vi "Open and close new editor.vi"(8 "error in (no error)":errorcluster) -> (0 "error out":errorcluster)   [LabVIEW 2013]
doc: "This vi is used to close 'Add device' editor and open 'Edit device' editor after adding device to database."
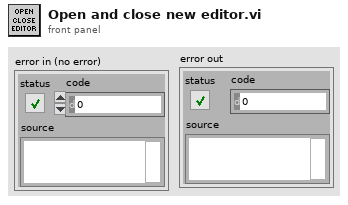
[diagram p1: front panel]
types:
  T1 = enum32{"invalid app kind", "Development System", "Run Time System", "Student Edition", "Embedded LabVIEW", "Evaluation", "Custom"}
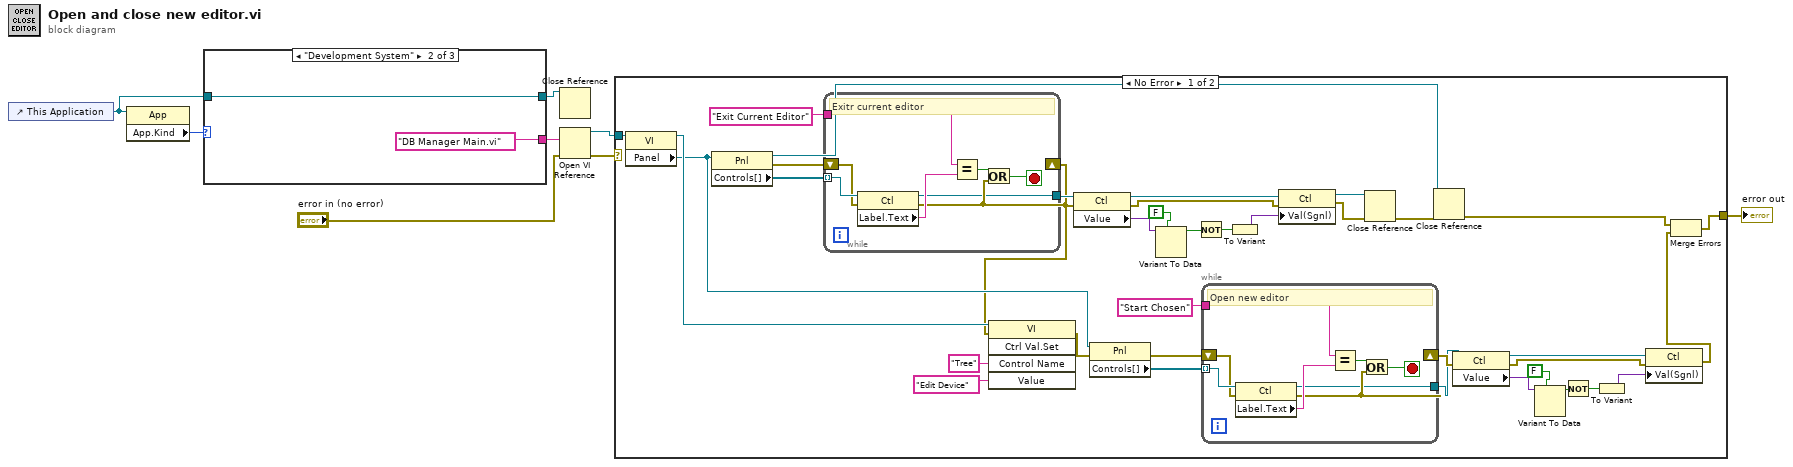
[diagram p0: block diagram]
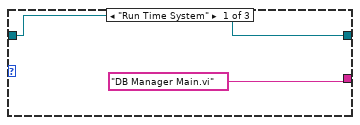
[diagram p2: hidden frame]
diagram:
  n1 = control-ref of="This Application"() -> (w2:refnum<vi>)
  n2 = property class="App"(reference=w2) -> ("App.Kind"=w3:T1)  [unwired: 1 in, 2 out]
  n3 = case shown="\"Development System\"" w3 {
    tunnel: ["DB Manager Main.vi" "DB Manager Main.vi" _] -> w8
    tunnel: w2 -> [w10 w12 w13]
    tunnel: [w10 w12 w13] -> w1
    frame "Run Time System" {
    }
    frame "Development System" {
    }
    frame "Student Edition", Default {
    }
  }
  n4 = Close Reference(reference=w1) -> ()  [unwired: 1 in, 1 out]
  n5 = Open VI Reference(vi path=w8, error in (no error)="error in (no error)") -> (vi reference=w7:refnum<vi>, error out=w5:errorcluster)  [unwired: 4 in]
  n6 = case shown="No Error" w5 {
    selector: w5 -> [_ w67]
    tunnel: w7 -> [w39 _]
    tunnel: [w14 w67] -> w4
    frame No Error {
      n7 = property class="VI"(reference=w39) -> (reference out=w38:refnum<vi>, "Panel"=w28:refnum<vi>)  [unwired: 1 in, 1 out]
      n8 = property class="Pnl"(reference=w28) -> (reference out=w41:refnum<vi>, error out=w40:errorcluster, "Controls[]"=w35:refnum<vi>[])  [unwired: 1 in]
      n9 = while {
        tunnel: w35 -> [w66] mode=indexing
        shift-right: [w60] -> w17
        shift-left: w40 -> [w65]
        tunnel: "Exit Current Editor" -> [w63]
        tunnel: [w59] -> w49
        stop <- w61 stop-if-true
        # "Exitr current editor"
        n10 = property class="Ctl"(reference=w66, error in=w65) -> (reference out=w59:refnum<vi>, error out=w60:errorcluster, "Label.Text"=w64:string)
        n11 = Equal?(x=w63, y=w64) -> (x = y?=w62:bool)
        n12 = Or(x=w62, y=w60) -> (x .or. y?=w61:bool)
      }
      n13 = invoke class="VI" method="Ctrl Val.Set"(reference=w38, error in=w17, "Control Name"="Tree", "Value"="Edit Device" ("Control Name")) -> (error out=w18:errorcluster)  [unwired: 1 in, 4 out]
      n14 = property class="Ctl"(reference=w49, error in=w17) -> (reference out=w43:refnum<vi>, error out=w33:errorcluster, "Value"=w48:variant)
      n15 = property class="Pnl"(reference=w28, error in=w18) -> (error out=w31:errorcluster, "Controls[]"=w32:refnum<vi>[])  [unwired: 1 out]
      n16 = Variant To Data(type=FALSE, Variant=w48) -> (data=w46:bool)  [unwired: 1 in, 1 out]
      n17 = Not(x=w46) -> (.not. x?=w45:bool)
      n18 = while {
        tunnel: w32 -> [w58] mode=indexing
        shift-right: [w52] -> w20
        shift-left: w31 -> [w57]
        tunnel: "Start Chosen" -> [w55]
        tunnel: [w51] -> w19
        stop <- w53 stop-if-true
        # "Open new editor"
        n19 = property class="Ctl"(reference=w58, error in=w57) -> (reference out=w51:refnum<vi>, error out=w52:errorcluster, "Label.Text"=w56:string)
        n20 = Equal?(x=w55, y=w56) -> (x = y?=w54:bool)
        n21 = Or(x=w54, y=w52) -> (x .or. y?=w53:bool)
      }
      n22 = To Variant(anything=w45) -> (Variant=w44:variant)
      n23 = property class="Ctl"(reference=w43, error in=w33, "Val(Sgnl)"=w44) -> (reference out=w42:refnum<vi>, error out=w29:errorcluster)
      n24 = Close Reference(reference=w42, error in (no error)=w29) -> (error out=w34:errorcluster)
      n25 = Close Reference(reference=w41, error in (no error)=w34) -> (error out=w15:errorcluster)
      n26 = property class="Ctl"(reference=w19, error in=w20) -> (reference out=w26:refnum<vi>, error out=w27:errorcluster, "Value"=w21:variant)
      n27 = Variant To Data(type=FALSE, Variant=w21) -> (data=w23:bool)  [unwired: 1 in, 1 out]
      n28 = Not(x=w23) -> (.not. x?=w24:bool)
      n29 = To Variant(anything=w24) -> (Variant=w25:variant)
      n30 = property class="Ctl"(reference=w26, error in=w27, "Val(Sgnl)"=w25) -> (error out=w16:errorcluster)  [unwired: 1 out]
      n31 = Merge Errors(w15, w16) -> (w14:errorcluster)
    }
    frame Error {
    }
  }
  "error out" <- w4
